vi "Servo Motor.vi"() -> ()   [LabVIEW 2020]
uses:
  Control 1.ctl
  <vilib>/DAQmx/create/channels.llb/DAQmx Create Channel (CO-Pulse Generation-Time).vi
  <vilib>/DAQmx/configure/timing.llb/DAQmx Timing (Implicit).vi
  <resource>/objmgr/daqmx.rc
panel:
  out "Cur Direction":bool
  in  "CO.Pulse.Term":tag
  out "High Width":dbl
  in  "Speed":cluster{"Slow":bool, "Medium":bool, "Fast":bool}
  in  "Direction":T1
  in  "stop":bool
  in  "Tab Control":enum32{"Finite Spin", "Countinuous Spin"}(tab)
  in  "Start Finite Spin":bool
  in  "Number of Pulses":i32
  in  "Start Continuous Spin":bool
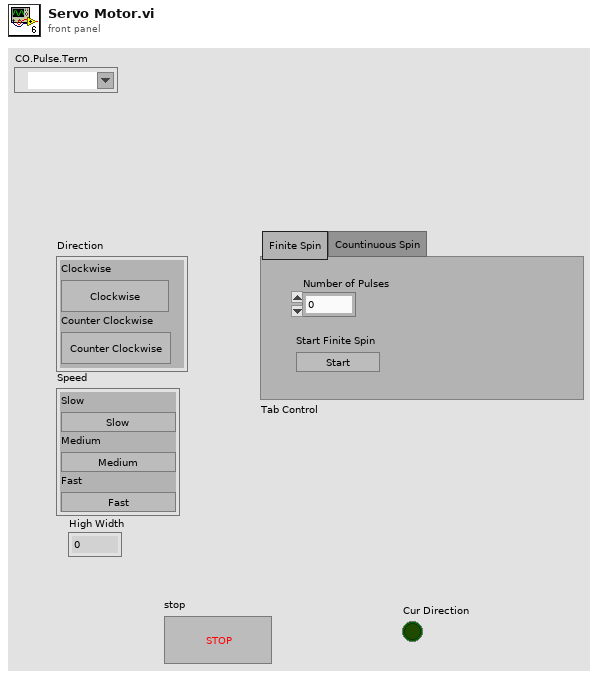
[diagram p1: front panel]
types:
  T1 = cluster{"Clockwise":bool, "Counter Clockwise":bool}
  T2 = typedef "Control 1.ctl" = enum16{"Init", "Wait for GUI", "Stop"}
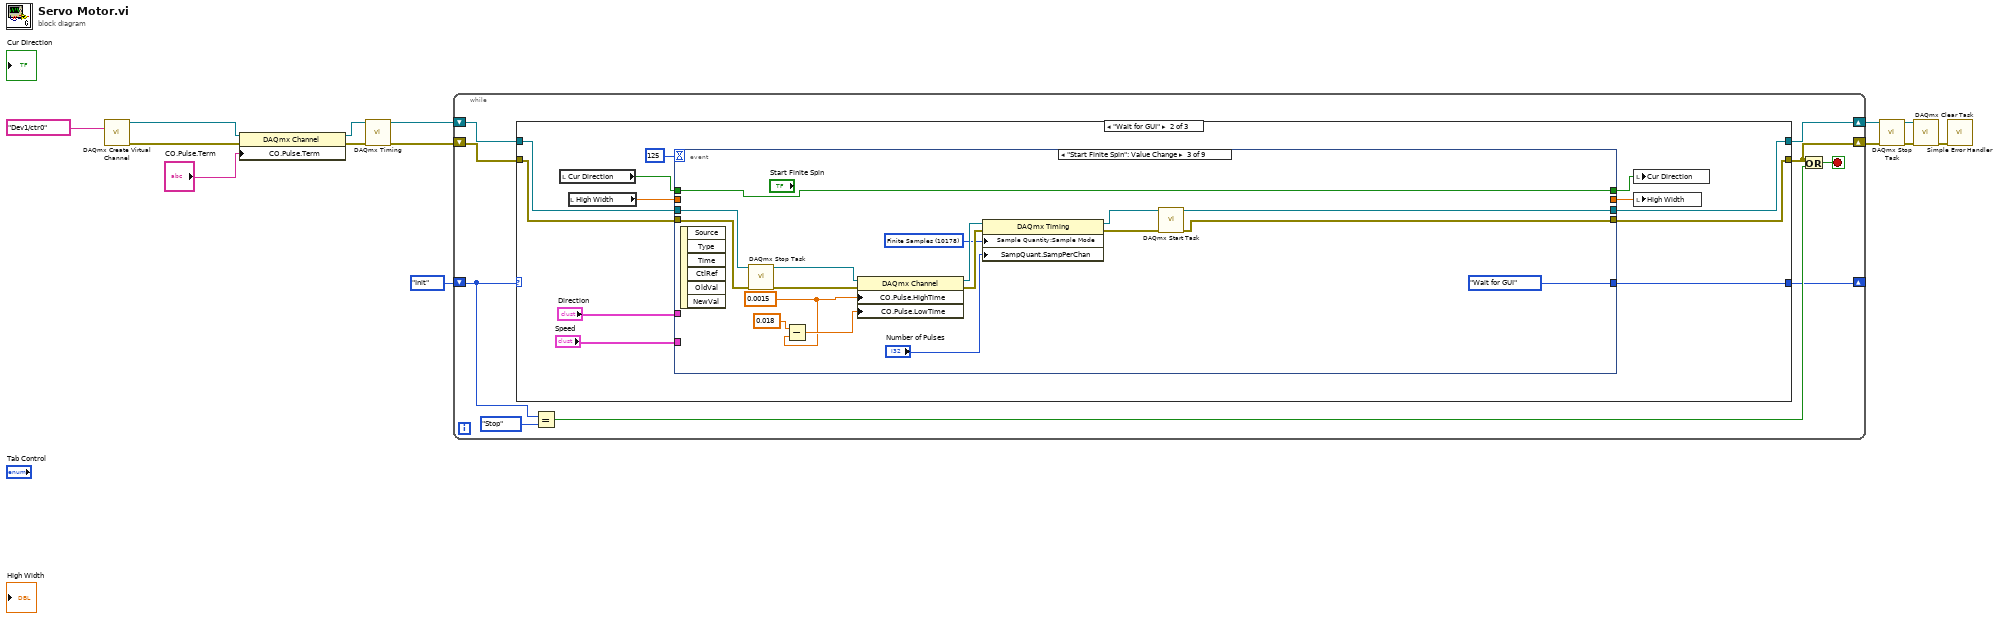
[diagram p0: block diagram]
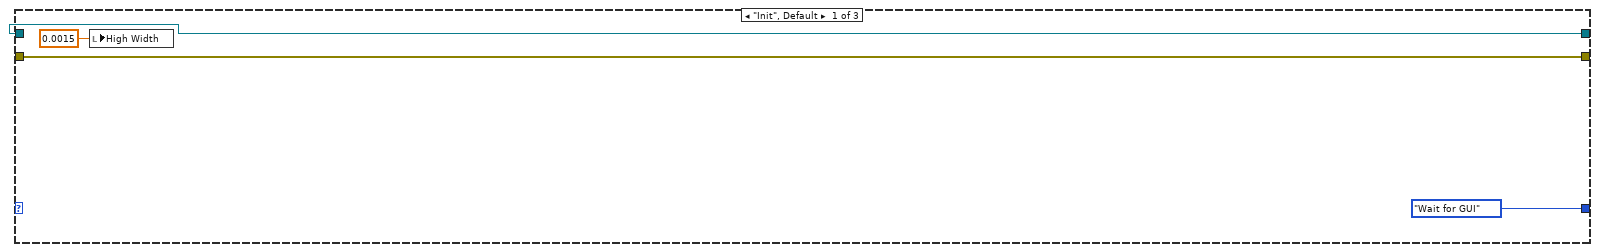
[diagram p2: hidden frame]
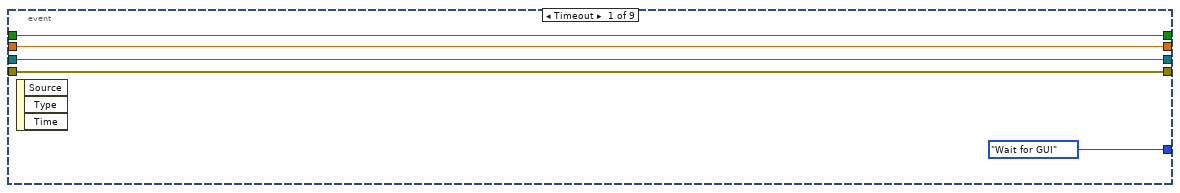
[diagram p3: hidden frame]
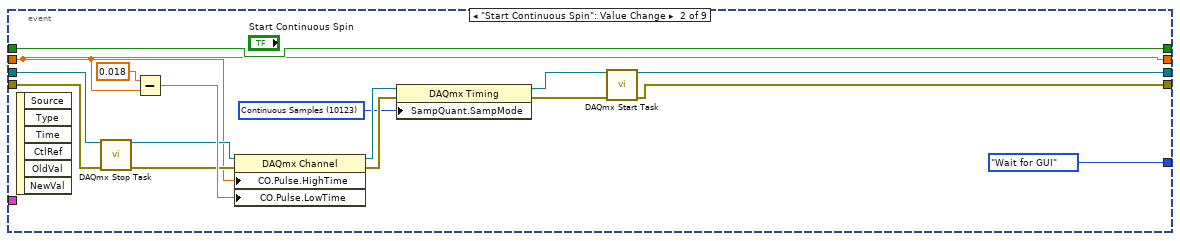
[diagram p4: hidden frame]
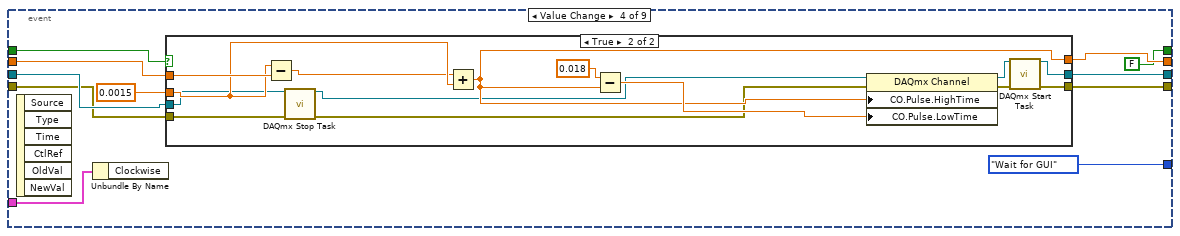
[diagram p5: hidden frame]
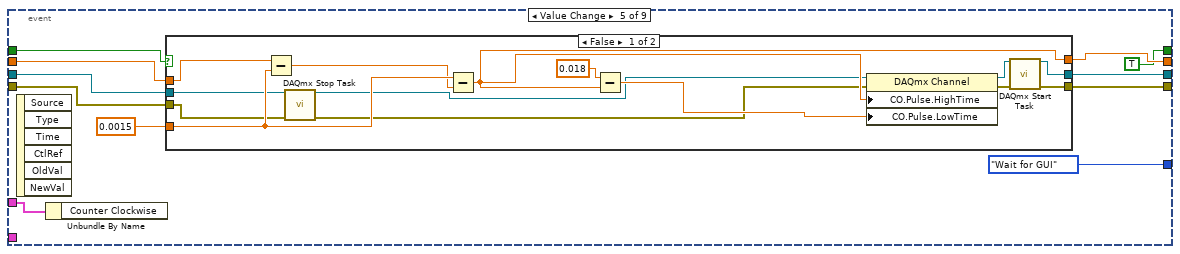
[diagram p7: hidden frame]
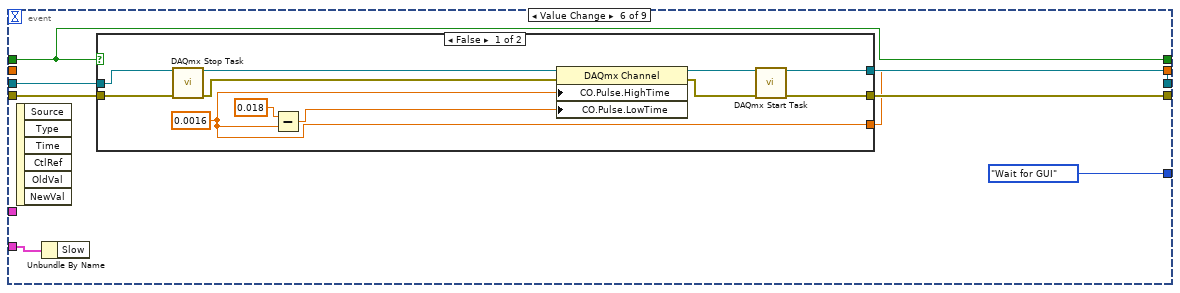
[diagram p9: hidden frame]
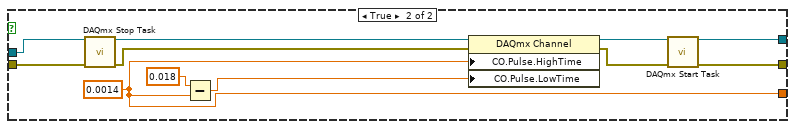
[diagram p10: hidden frame]
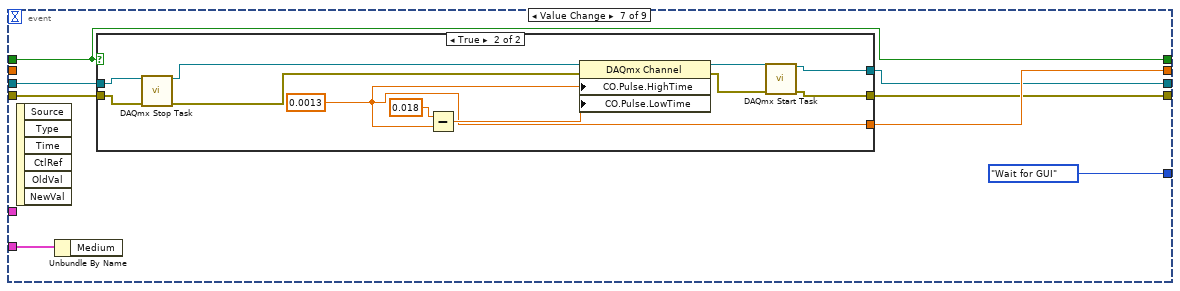
[diagram p11: hidden frame]
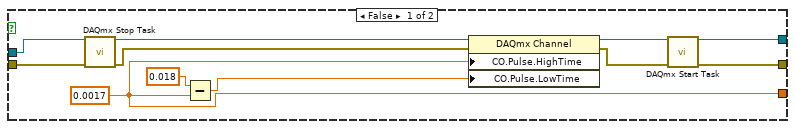
[diagram p12: hidden frame]
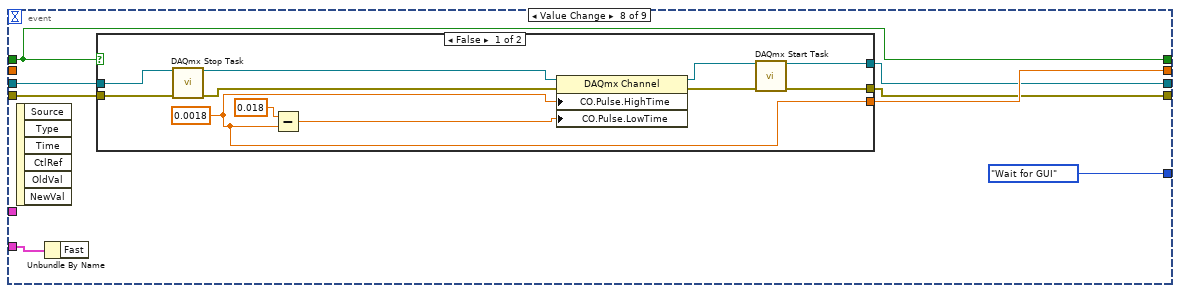
[diagram p13: hidden frame]
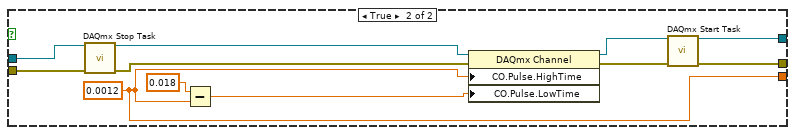
[diagram p14: hidden frame]
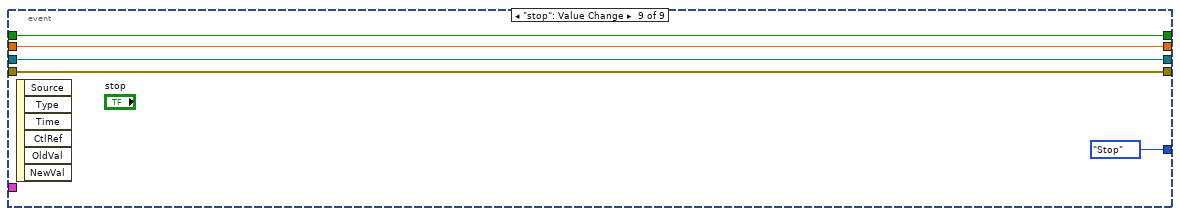
[diagram p15: hidden frame]
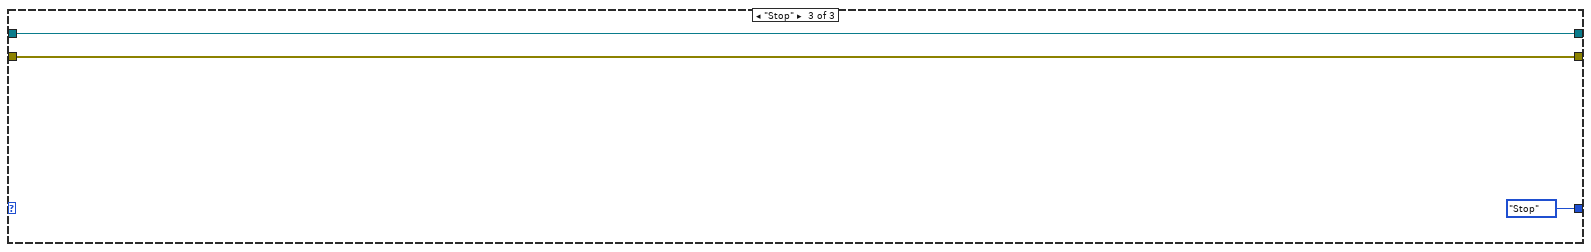
[diagram p16: hidden frame]
diagram:
  n1 = call-poly <vilib>:"DAQmx Create Virtual Channel.vi"("counter"=tag "Dev1/ctr0") -> ("task out"=w12:refnum<k21>, "error out"=w11:errorcluster)  [unwired: 13 in]
  n2 = property class="DAQmx Channel"(reference=w12, error in=w11, "CO.Pulse.Term"="CO.Pulse.Term") -> (reference out=w4:refnum<k21>, error out=w3:errorcluster)
  n3 = call-poly <vilib>:"DAQmx Timing.vi"("task/channels in"=w4, "error in"=w3) -> ("task out"=w2:refnum<k21>, "error out"=w1:errorcluster)  [unwired: 12 in]
  n4 = while {
    shift-right: [w17] -> _
    shift-left: Control_1."Init" -> [w18]
    shift-right: [w23] -> w6
    shift-left: w2 -> [w16]
    shift-right: [w22] -> w5
    shift-left: w1 -> [w15]
    stop <- w20 stop-if-true
    n5 = case shown="\"Wait for GUI\"" w18 {
      tunnel: w16 -> [w26 w39 w231]
      tunnel: w15 -> [w25 w38 w230]
      tunnel: [w26 w37 w231] -> w23
      tunnel: [w25 w36 w230] -> w22
      tunnel: [Control_1."Wait for GUI" w30 Control_1."Stop"] -> w17
      frame "Init", Default {
        n6 = local write "High Width"(0.0015 ("High Width")) -> ()
      }
      frame "Wait for GUI" {
        n7 = local read "Cur Direction"() -> (w31:bool)
        n8 = local read "High Width"() -> (w34:dbl)
        n9 = event shown="[2] \"Start Finite Spin\": Value Change" {
          selector: _ -> [_ _ _ _ _ _ _ _ _]
          dyn-events: _ -> [_ _ _ _ _ _ _ _ _]
          timeout: 125 -> [_ _ _ _ _ _ _ _ _]
          tunnel: w39 -> [w44 w49 w65 w83 w110 w141 w169 w198 w227]
          tunnel: w38 -> [w43 w48 w64 w82 w109 w140 w168 w199 w226]
          tunnel: [w44 w54 w72 w80 w108 w139 w167 w197 w227] -> w37
          tunnel: [w43 w53 w71 w79 w107 w138 w166 w196 w226] -> w36
          tunnel: w34 -> [w42 w45 _ w88 w111 _ _ _ w225]
          tunnel: [w42 w45 _ w87 w115 w137 w170 w200 w225] -> w33
          tunnel: [w41 w51 w67 FALSE TRUE w136 w171 w201 w224] -> w32
          tunnel: w31 -> [w41 w51 w67 w84 w112 w136 w171 w201 w224]
          tunnel: [Control_1."Wait for GUI" Control_1."Wait for GUI" Control_1."Wait for GUI" Control_1."Wait for GUI" Control_1."Wait for GUI" Control_1."Wait for GUI" Control_1."Wait for GUI" Control_1."Wait for GUI" Control_1."Stop"] -> w30
          tunnel: "Direction" -> [_ _ _ w78 w106 _ _ _ _]
          tunnel: "Speed" -> [_ _ _ _ _ w134 w164 w194 _]
          event Timeout {
            n10 = event-data() -> ()  [unwired: 1 in, 3 out]
          }
          event "Start Continuous Spin": Value Change {
            w55 = 10123 items=["Finite Samples"=10178, "Continuous Samples"=10123, "Hardware Timed Single Point"=12522] ("SampQuant.SampMode")
            n11 = event-data() -> ()  [unwired: 1 in, 6 out]
            n12 = call <vilib>:"DAQmx Stop Task.vi"("task/channels in"=w49, "error in"=w48) -> ("task out"=w47:refnum<k21>, "error out"=w46:errorcluster)  [unwired: 12 in]
            n13 = Subtract(x=0.018, y=w45) -> (x-y=w52:dbl)
            n14 = property class="DAQmx Channel"(reference=w47, error in=w46, "CO.Pulse.HighTime"=w45, "CO.Pulse.LowTime"=w52) -> (reference out=w59:refnum<k21>, error out=w58:errorcluster)
            n15 = property class="DAQmx Timing"(reference=w59, error in=w58, "SampQuant.SampMode"=w55) -> (reference out=w57:refnum<k21>, error out=w56:errorcluster)
            n16 = call <vilib>:"DAQmx Start Task.vi"("task/channels in"=w57, "error in"=w56) -> ("task out"=w54:refnum<k21>, "error out"=w53:errorcluster)  [unwired: 12 in]
          }
          event "Start Finite Spin": Value Change {
            w61 = 0.0015 ("CO.Pulse.HighTime")
            w74 = 10178 items=["Finite Samples"=10178, "Continuous Samples"=10123, "Hardware Timed Single Point"=12522] ("SampQuant.SampMode")
            n17 = event-data() -> ()  [unwired: 1 in, 6 out]
            n18 = call <vilib>:"DAQmx Stop Task.vi"("task/channels in"=w65, "error in"=w64) -> ("task out"=w63:refnum<k21>, "error out"=w62:errorcluster)  [unwired: 12 in]
            n19 = Subtract(x=0.018, y=w61) -> (x-y=w68:dbl)
            n20 = property class="DAQmx Channel"(reference=w63, error in=w62, "CO.Pulse.HighTime"=w61, "CO.Pulse.LowTime"=w68) -> (reference out=w76:refnum<k21>, error out=w75:errorcluster)
            n21 = property class="DAQmx Timing"(reference=w76, error in=w75, "Sample Quantity:Sample Mode"=w74, "SampQuant.SampPerChan"="Number of Pulses") -> (reference out=w70:refnum<k21>, error out=w69:errorcluster)
            n22 = call <vilib>:"DAQmx Start Task.vi"("task/channels in"=w70, "error in"=w69) -> ("task out"=w72:refnum<k21>, "error out"=w71:errorcluster)  [unwired: 12 in]
          }
          event "Direction.Clockwise": Value Change {
            n23 = event-data() -> ()  [unwired: 1 in, 6 out]
            n24 = Unbundle By Name(w78) -> ()  [unwired: 1 out]
            n25 = case shown="True" w84 {
              tunnel: 0.0015 ("y") -> [_ w104]
              tunnel: w88 -> [w91 w105]
              tunnel: [w91 w100] -> w87
              tunnel: w83 -> [w90 w95]
              tunnel: w82 -> [w89 w94]
              tunnel: [w90 w97] -> w80
              tunnel: [w89 w96] -> w79
              frame False {
              }
              frame True {
                n26 = Subtract(x=w104, y=w105) -> (x-y=w103:dbl)
                n27 = call <vilib>:"DAQmx Stop Task.vi"("task/channels in"=w95, "error in"=w94) -> ("task out"=w93:refnum<k21>, "error out"=w92:errorcluster)  [unwired: 12 in]
                n28 = Add(x=w103, y=w104) -> (x+y=w100:dbl)
                n29 = Subtract(x=0.018, y=w100) -> (x-y=w102:dbl)
                n30 = property class="DAQmx Channel"(reference=w93, error in=w92, "CO.Pulse.HighTime"=w100, "CO.Pulse.LowTime"=w102) -> (reference out=w99:refnum<k21>, error out=w98:errorcluster)
                n31 = call <vilib>:"DAQmx Start Task.vi"("task/channels in"=w99, "error in"=w98) -> ("task out"=w97:refnum<k21>, "error out"=w96:errorcluster)  [unwired: 12 in]
              }
            }
          }
          event "Direction.Counter Clockwise": Value Change {
            n32 = event-data() -> ()  [unwired: 1 in, 6 out]
            n33 = Unbundle By Name(w106) -> ()  [unwired: 1 out]
            n34 = case shown="False" w112 {
              tunnel: 0.0015 ("y") -> [w129 _]
              tunnel: [w125 w133] -> w115
              tunnel: w111 -> [w130 w133]
              tunnel: w110 -> [w127 w132]
              tunnel: w109 -> [w126 w131]
              tunnel: [w118 w132] -> w108
              tunnel: [w117 w131] -> w107
              frame False {
                n35 = Subtract(x=w130, y=w129) -> (x-y=w128:dbl)
                n36 = call <vilib>:"DAQmx Stop Task.vi"("task/channels in"=w127, "error in"=w126) -> ("task out"=w122:refnum<k21>, "error out"=w121:errorcluster)  [unwired: 12 in]
                n37 = Subtract(x=w129, y=w128) -> (x-y=w125:dbl)
                n38 = Subtract(x=0.018, y=w125) -> (x-y=w123:dbl)
                n39 = property class="DAQmx Channel"(reference=w122, error in=w121, "CO.Pulse.HighTime"=w125, "CO.Pulse.LowTime"=w123) -> (reference out=w120:refnum<k21>, error out=w119:errorcluster)
                n40 = call <vilib>:"DAQmx Start Task.vi"("task/channels in"=w120, "error in"=w119) -> ("task out"=w118:refnum<k21>, "error out"=w117:errorcluster)  [unwired: 12 in]
              }
              frame True {
              }
            }
          }
          event "Speed.Slow": Value Change {
            n41 = event-data() -> ()  [unwired: 1 in, 6 out]
            n42 = Unbundle By Name(w134) -> ()  [unwired: 1 out]
            n43 = case shown="False" w136 {
              tunnel: w141 -> [w149 w160]
              tunnel: w140 -> [w148 w159]
              tunnel: [w143 w154] -> w139
              tunnel: [w142 w153] -> w138
              tunnel: [w150 w161] -> w137
              frame False {
                w150 = 0.0016 ("CO.Pulse.HighTime")
                n44 = call <vilib>:"DAQmx Stop Task.vi"("task/channels in"=w149, "error in"=w148) -> ("task out"=w147:refnum<k21>, "error out"=w146:errorcluster)  [unwired: 12 in]
                n45 = Subtract(x=0.018, y=w150) -> (x-y=w151:dbl)
                n46 = property class="DAQmx Channel"(reference=w147, error in=w146, "CO.Pulse.HighTime"=w150, "CO.Pulse.LowTime"=w151) -> (reference out=w145:refnum<k21>, error out=w144:errorcluster)
                n47 = call <vilib>:"DAQmx Start Task.vi"("task/channels in"=w145, "error in"=w144) -> ("task out"=w143:refnum<k21>, "error out"=w142:errorcluster)  [unwired: 12 in]
              }
              frame True {
                w161 = 0.0014 ("CO.Pulse.HighTime")
                n48 = call <vilib>:"DAQmx Stop Task.vi"("task/channels in"=w160, "error in"=w159) -> ("task out"=w158:refnum<k21>, "error out"=w157:errorcluster)  [unwired: 12 in]
                n49 = Subtract(x=0.018, y=w161) -> (x-y=w162:dbl)
                n50 = property class="DAQmx Channel"(reference=w158, error in=w157, "CO.Pulse.HighTime"=w161, "CO.Pulse.LowTime"=w162) -> (reference out=w156:refnum<k21>, error out=w155:errorcluster)
                n51 = call <vilib>:"DAQmx Start Task.vi"("task/channels in"=w156, "error in"=w155) -> ("task out"=w154:refnum<k21>, "error out"=w153:errorcluster)  [unwired: 12 in]
              }
            }
          }
          event "Speed.Medium": Value Change {
            n52 = event-data() -> ()  [unwired: 1 in, 6 out]
            n53 = Unbundle By Name(w164) -> ()  [unwired: 1 out]
            n54 = case shown="True" w171 {
              tunnel: w169 -> [w179 w190]
              tunnel: w168 -> [w178 w189]
              tunnel: [w173 w184] -> w167
              tunnel: [w172 w183] -> w166
              tunnel: [w180 w191] -> w170
              frame False {
                w180 = 0.0017 ("CO.Pulse.HighTime")
                n55 = call <vilib>:"DAQmx Stop Task.vi"("task/channels in"=w179, "error in"=w178) -> ("task out"=w177:refnum<k21>, "error out"=w176:errorcluster)  [unwired: 12 in]
                n56 = Subtract(x=0.018, y=w180) -> (x-y=w181:dbl)
                n57 = property class="DAQmx Channel"(reference=w177, error in=w176, "CO.Pulse.HighTime"=w180, "CO.Pulse.LowTime"=w181) -> (reference out=w175:refnum<k21>, error out=w174:errorcluster)
                n58 = call <vilib>:"DAQmx Start Task.vi"("task/channels in"=w175, "error in"=w174) -> ("task out"=w173:refnum<k21>, "error out"=w172:errorcluster)  [unwired: 12 in]
              }
              frame True {
                w191 = 0.0013 ("CO.Pulse.HighTime")
                n59 = call <vilib>:"DAQmx Stop Task.vi"("task/channels in"=w190, "error in"=w189) -> ("task out"=w188:refnum<k21>, "error out"=w187:errorcluster)  [unwired: 12 in]
                n60 = Subtract(x=0.018, y=w191) -> (x-y=w192:dbl)
                n61 = property class="DAQmx Channel"(reference=w188, error in=w187, "CO.Pulse.HighTime"=w191, "CO.Pulse.LowTime"=w192) -> (reference out=w186:refnum<k21>, error out=w185:errorcluster)
                n62 = call <vilib>:"DAQmx Start Task.vi"("task/channels in"=w186, "error in"=w185) -> ("task out"=w184:refnum<k21>, "error out"=w183:errorcluster)  [unwired: 12 in]
              }
            }
          }
          event "Speed.Fast": Value Change {
            n63 = event-data() -> ()  [unwired: 1 in, 6 out]
            n64 = Unbundle By Name(w194) -> ()  [unwired: 1 out]
            n65 = case shown="False" w201 {
              tunnel: w198 -> [w203 w214]
              tunnel: w199 -> [w202 w213]
              tunnel: [w205 w218] -> w197
              tunnel: [w204 w217] -> w196
              tunnel: [w210 w221] -> w200
              frame False {
                w210 = 0.0018 ("CO.Pulse.HighTime")
                n66 = call <vilib>:"DAQmx Stop Task.vi"("task/channels in"=w203, "error in"=w202) -> ("task out"=w209:refnum<k21>, "error out"=w208:errorcluster)  [unwired: 12 in]
                n67 = Subtract(x=0.018, y=w210) -> (x-y=w211:dbl)
                n68 = property class="DAQmx Channel"(reference=w209, error in=w208, "CO.Pulse.HighTime"=w210, "CO.Pulse.LowTime"=w211) -> (reference out=w207:refnum<k21>, error out=w206:errorcluster)
                n69 = call <vilib>:"DAQmx Start Task.vi"("task/channels in"=w207, "error in"=w206) -> ("task out"=w205:refnum<k21>, "error out"=w204:errorcluster)  [unwired: 12 in]
              }
              frame True {
                w221 = 0.0012 ("CO.Pulse.HighTime")
                n70 = call <vilib>:"DAQmx Stop Task.vi"("task/channels in"=w214, "error in"=w213) -> ("task out"=w216:refnum<k21>, "error out"=w215:errorcluster)  [unwired: 12 in]
                n71 = Subtract(x=0.018, y=w221) -> (x-y=w222:dbl)
                n72 = property class="DAQmx Channel"(reference=w216, error in=w215, "CO.Pulse.HighTime"=w221, "CO.Pulse.LowTime"=w222) -> (reference out=w220:refnum<k21>, error out=w219:errorcluster)
                n73 = call <vilib>:"DAQmx Start Task.vi"("task/channels in"=w220, "error in"=w219) -> ("task out"=w218:refnum<k21>, "error out"=w217:errorcluster)  [unwired: 12 in]
              }
            }
          }
          event "stop": Value Change {
            n74 = event-data() -> ()  [unwired: 1 in, 6 out]
          }
        }
        n75 = local write "Cur Direction"(w32) -> ()
        n76 = local write "High Width"(w33) -> ()
      }
      frame "Stop" {
      }
    }
    n77 = Equal?(x=w18, y=Control_1."Stop") -> (x = y?=w21:bool)
    n78 = Or(x=w22, y=w21) -> (x .or. y?=w20:bool)
  }
  n79 = call <vilib>:"DAQmx Stop Task.vi"("task/channels in"=w6, "error in"=w5) -> ("task out"=w7:refnum<k21>, "error out"=w8:errorcluster)  [unwired: 12 in]
  n80 = call <vilib>:"DAQmx Clear Task.vi"("task in"=w7, "error in"=w8) -> ("error out"=w9:errorcluster)  [unwired: 13 in]
  n81 = call <vilib>:"Simple Error Handler.vi"("error in (no error)"=w9) -> ()  [unwired: 4 in, 5 out]
